vi "CCD spectrum processing_Shaowei-v4.vi"() -> ()   [LabVIEW 2012]
uses:
  <vilib>/Utility/file.llb/Read From Spreadsheet File (DBL).vi
panel:
  in  "save 2":bool
  in  "save 1":bool
  in  "select 2":bool
  in  "select":bool
  in  "next 2":bool
  in  "next":bool
  in  "previous 2":bool
  in  "previous":bool
  in  "Do it":bool
  out "?":path
  out "?":path
  out "Spec2 File name":string
  out "Spec1 File name":string
  in  "window switch":bool
  out "Spectrum 2":cluster{"Y":dbl[], "Y":dbl[]}[](graph)
  in  "?":bool=TRUE
  in  "?":bool
  out "Y":sgl
  out "X":sgl
  out "MIN":dbl
  out "MAX":dbl
  out "Spectrum 1":cluster{"Y":dbl[], "Y":dbl[]}[](graph)
  in  "file switch":bool
  out "?":ext=1340.0
  in  "cosmic ray removal":bool
  in  "?":i32(ring)=1 items=["nm"=1, "eV"=2, "cm-1"=3, "Pixel #"=4]
  # "Input File"
  # "1 File"
  # "2 Files"
  # "1st"
  # "2nd"
  # "Active Window"
  # "#1"
  # "#2"
  # "Save As"
  # "# of Pixel"
  # "X unit"
  # "Cosmic Ray Removal"
  # "NO"
  # "YES"
  # "Value"
  # "Position"
  # "Output Setting"
  # "Descending"
  # "Sort Data by X"
  # "Save As"
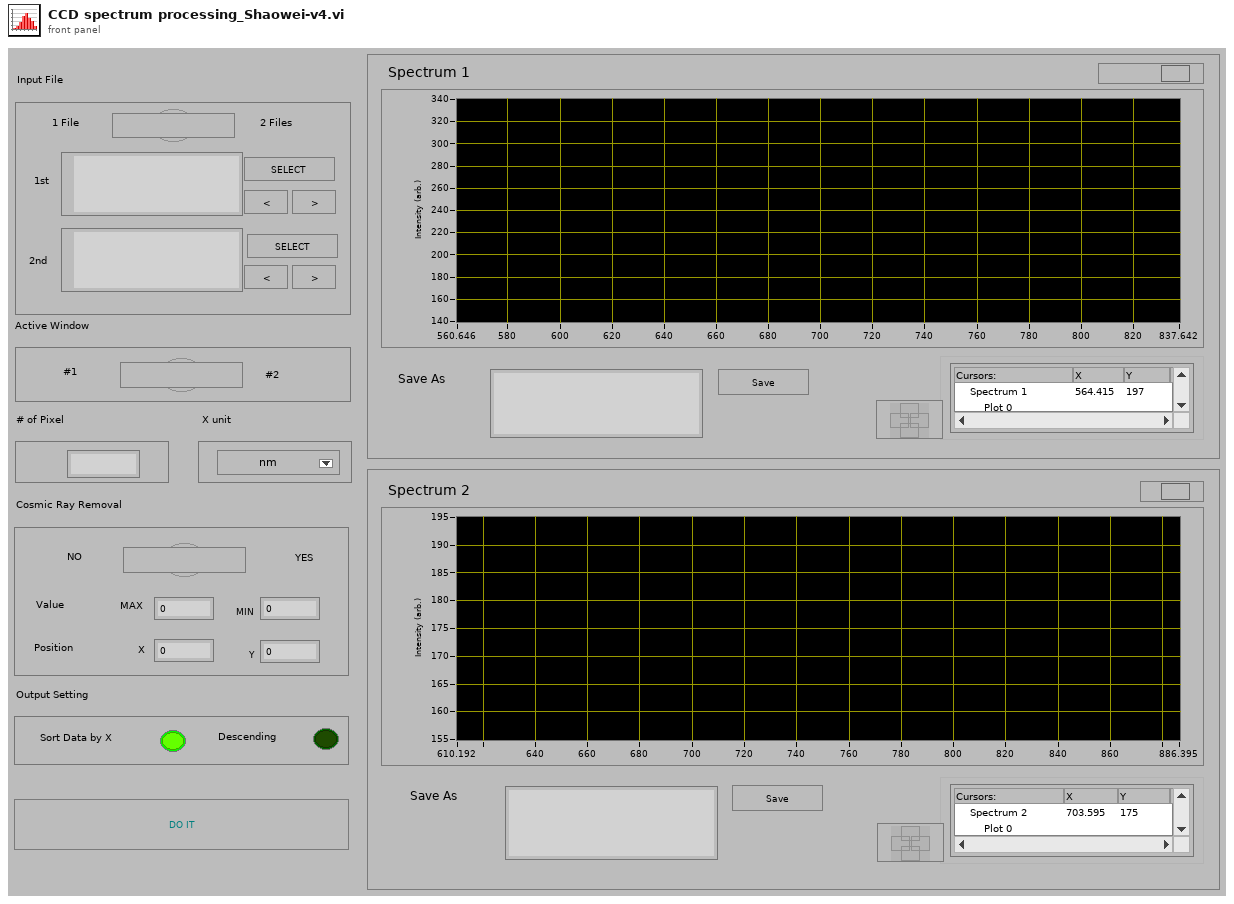
[diagram p1: front panel]
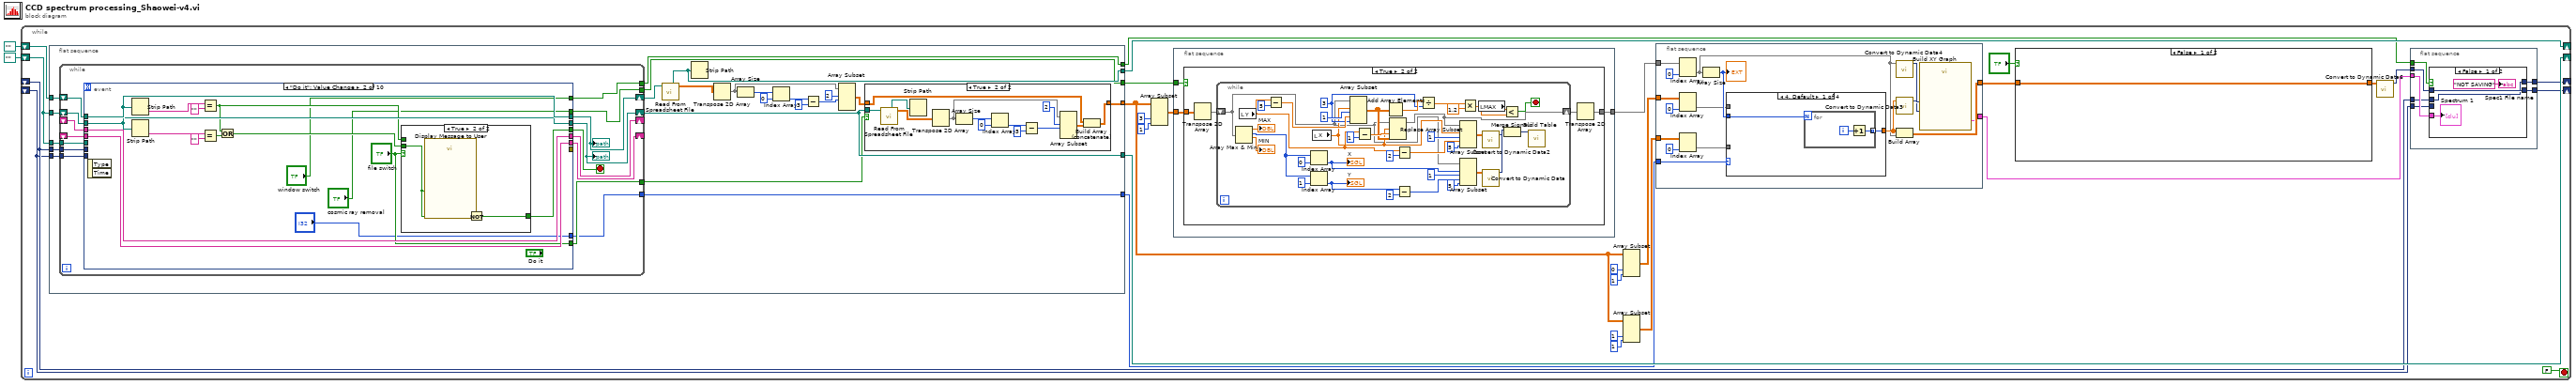
[diagram p0: block diagram]
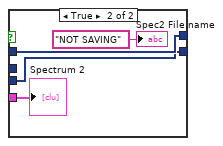
[diagram p2: hidden frame]
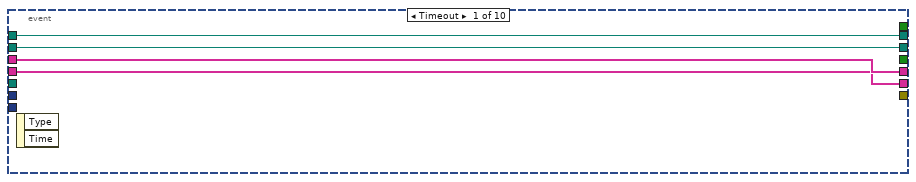
[diagram p3: hidden frame]
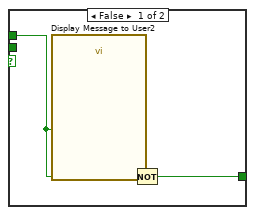
[diagram p4: hidden frame]
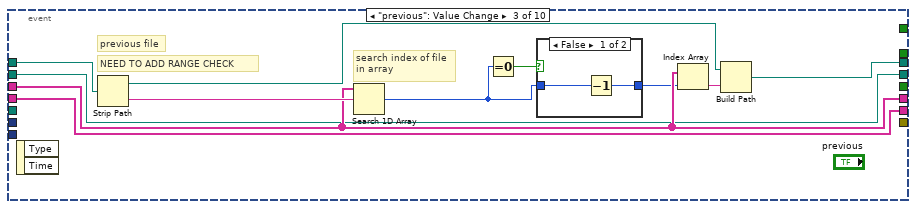
[diagram p5: hidden frame]
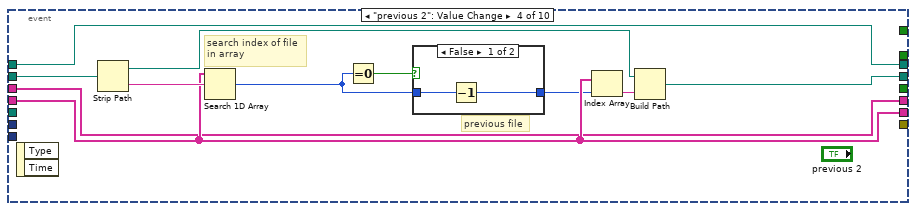
[diagram p7: hidden frame]
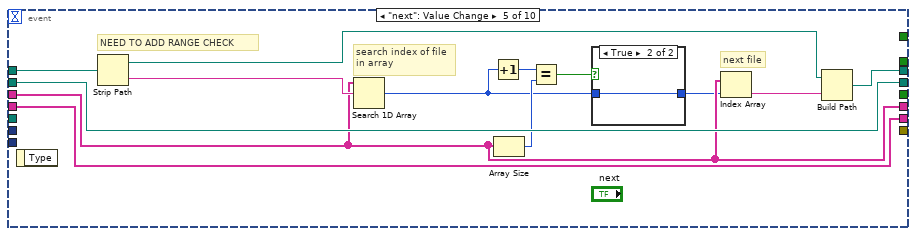
[diagram p9: hidden frame]
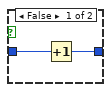
[diagram p10: hidden frame]
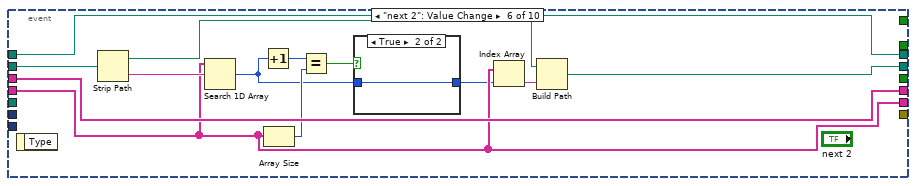
[diagram p11: hidden frame]
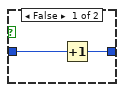
[diagram p12: hidden frame]
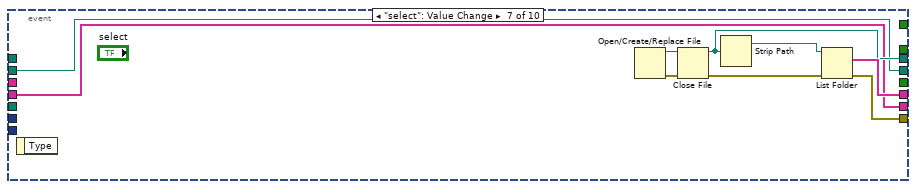
[diagram p13: hidden frame]
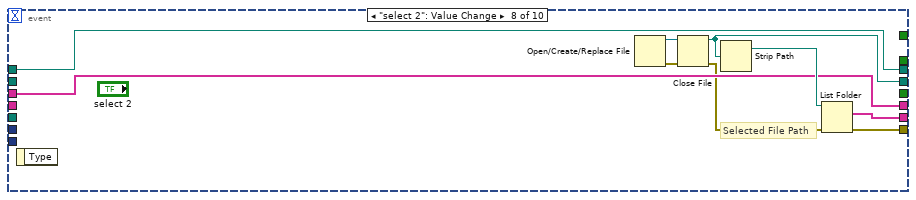
[diagram p14: hidden frame]
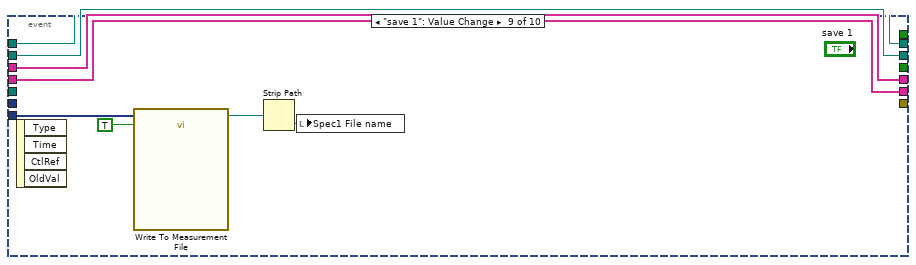
[diagram p15: hidden frame]
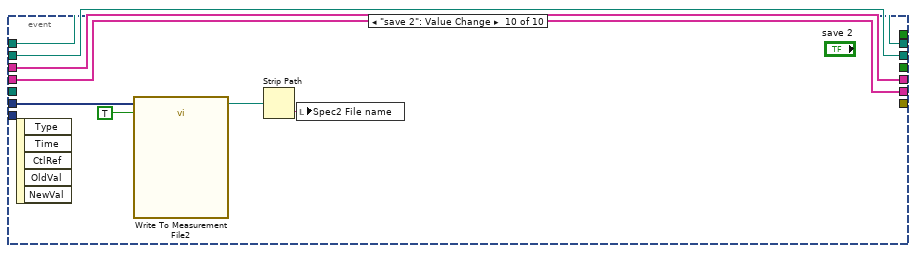
[diagram p16: hidden frame]
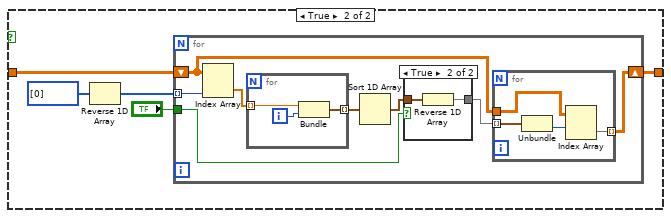
[diagram p18: hidden frame]
diagram:
  n1 = while {
    shift-right: [w22] -> _
    shift-left: path "" ("new file path (Not A Path if cancelled)") -> [w23]
    shift-right: [w21] -> _
    shift-left: path "" ("path") -> [w3]
    shift-right: [w7] -> _
    shift-left: _ -> [w4]
    shift-right: [w6] -> _
    shift-left: _ -> [w5]
    stop <- FALSE ("stop 2") stop-if-true
    n2 = flat-sequence {
      tunnel: [w66] -> w10
      tunnel: w23 -> [w64]
      tunnel: w3 -> [w63]
      tunnel: [w62] -> w22
      tunnel: [w61] -> w21
      tunnel: [w59] -> w20
      tunnel: [w58] -> w19
      tunnel: [w57] -> w18
      tunnel: w5 -> [w56]
      tunnel: w4 -> [w55]
      tunnel: w3 -> [w46]
      frame #0 {
        n3 = while {
          shift-right: [w82] -> _
          shift-left: _ -> [w81]
          shift-right: [w83] -> w65
          shift-left: w64 -> [w80]
          shift-right: [w79] -> w61
          shift-left: w63 -> [w78]
          shift-right: [w77] -> _
          shift-left: _ -> [w76]
          tunnel: [w71] -> w60
          tunnel: [w69] -> w59
          tunnel: [w68] -> w58
          tunnel: [w70] -> w57
          tunnel: w56 -> [w74]
          tunnel: w55 -> [w73]
          tunnel: w46 -> [w72]
          stop <- w75 stop-if-true
          n4 = event shown="[1] \"Do it\": Value Change" {
            selector: _ -> [_ _ _ _ _ _ _ _ _ _]
            dyn-events: _ -> [_ _ _ _ _ _ _ _ _ _]
            timeout: _ -> [_ _ _ _ _ _ _ _ _ _]
            tunnel: [_ w95 _ _ _ _ _ _ _ _] -> w75
            tunnel: [w86 w101 w113 w122 w145 w153 w173 w181 w193 w201] -> w83
            tunnel: [w87 w103 w115 w127 w138 w161 w174 w180 w192 w200] -> w82
            tunnel: w81 -> [w87 w103 w115 w127 w138 w161 _ w180 w192 w200]
            tunnel: w80 -> [w86 w101 w118 w122 w144 w153 _ w181 w193 w201]
            tunnel: [w84 w96 w111 w123 w142 w154 w171 w183 w187 w196] -> w79
            tunnel: w78 -> [w84 w96 w111 w129 w142 w152 w171 _ w187 w196]
            tunnel: [w85 w102 w112 w128 w143 w157 w172 w182 w188 w197] -> w77
            tunnel: w76 -> [w85 w102 w112 w128 w143 w157 w172 _ w188 w197]
            tunnel: [_ _ _ _ _ _ w168 w177 _ _] -> _
            tunnel: w74 -> [_ _ _ _ _ _ _ _ _ w194]
            tunnel: w73 -> [_ _ _ _ _ _ _ _ w186 _]
            tunnel: w72 -> [_ _ _ _ _ _ _ _ _ _]
            tunnel: [_ "file switch" _ _ _ _ _ _ _ _] -> w71
            tunnel: [_ "window switch" _ _ _ _ _ _ _ _] -> w70
            tunnel: [_ "cosmic ray removal" _ _ _ _ _ _ _ _] -> w69
            tunnel: [_ "?" _ _ _ _ _ _ _ _] -> w68
            event Timeout {
              n5 = event-data() -> ()  [unwired: 1 in, 2 out]
            }
            event "Do it": Value Change {
              n6 = event-data() -> ()  [unwired: 1 in, 2 out]
              n7 = Strip Path(path=w101) -> (name=w100:string)  [unwired: 1 out]
              n8 = Strip Path(path=w96) -> (name=w98:string)  [unwired: 1 out]
              n9 = Equal?(x=w100, y="") -> (x = y?=w94:bool)
              n10 = Equal?(x=w98, y="") -> (x = y?=w93:bool)
              n11 = Or(x=w94, y=w93) -> (x .or. y?=w92:bool)
              n12 = case shown="True" "file switch" {
                tunnel: w94 -> [w104 _]
                tunnel: [w105 w107] -> w95
                tunnel: w92 -> [_ w106]
                frame False {
                  n13 = call "Display Message to User2"("Enable"=w104) -> ()  [unwired: 9 in, 2 out]
                  n14 = Not(x=w104) -> (.not. x?=w105:bool)
                }
                frame True {
                  n15 = call "Display Message to User"("Enable"=w106) -> ()  [unwired: 9 in, 2 out]
                  n16 = Not(x=w106) -> (.not. x?=w107:bool)
                }
              }
            }
            event "previous": Value Change {
              # "NEED TO ADD RANGE CHECK"
              # "previous file"
              # "search index of file\nin array"
              n17 = event-data() -> ()  [unwired: 1 in, 2 out]
              n18 = Strip Path(path=w118) -> (stripped path=w116:path, name=w117:string)
              n19 = Search 1D Array(1D array=w115, element=w117) -> (index of element=w109:i32)  [unwired: 1 in]
              n20 = Equal To 0?(x=w109) -> (x = 0?=w110:bool)
              n21 = case shown="False" w110 {
                tunnel: w109 -> [w120 w121]
                tunnel: [w119 w121] -> w108
                frame False {
                  n22 = Decrement(x=w120) -> (x-1=w119:i32)
                }
                frame True {
                }
              }
              n23 = Index Array(array=w115, index=w108) -> (element=w114:string)
              n24 = Build Path(base path=w116, name or relative path=w114) -> (appended path=w113:path)
            }
            event "previous 2": Value Change {
              # "previous file"
              # "search index of file\nin array"
              n25 = event-data() -> ()  [unwired: 1 in, 2 out]
              n26 = Strip Path(path=w129) -> (stripped path=w131:path, name=w132:string)
              n27 = Search 1D Array(1D array=w128, element=w132) -> (index of element=w125:i32)  [unwired: 1 in]
              n28 = Equal To 0?(x=w125) -> (x = 0?=w126:bool)
              n29 = case shown="False" w126 {
                tunnel: w125 -> [w134 w135]
                tunnel: [w133 w135] -> w124
                frame False {
                  n30 = Decrement(x=w134) -> (x-1=w133:i32)
                }
                frame True {
                }
              }
              n31 = Index Array(array=w128, index=w124) -> (element=w130:string)
              n32 = Build Path(base path=w131, name or relative path=w130) -> (appended path=w123:path)
            }
            event "next": Value Change {
              # "NEED TO ADD RANGE CHECK"
              # "next file"
              # "search index of file\nin array"
              n33 = event-data() -> ()  [unwired: 1 in, 1 out]
              n34 = Strip Path(path=w144) -> (stripped path=w147:path, name=w148:string)
              n35 = Search 1D Array(1D array=w138, element=w148) -> (index of element=w137:i32)  [unwired: 1 in]
              n36 = Increment(x=w137) -> (x+1=w139:i32)
              n37 = Array Size(array=w138) -> (size(s)=w141:i32)
              n38 = Equal?(x=w139, y=w141) -> (x = y?=w140:bool)
              n39 = case shown="True" w140 {
                tunnel: w137 -> [w150 w151]
                tunnel: [w149 w151] -> w136
                frame False {
                  n40 = Increment(x=w150) -> (x+1=w149:i32)
                }
                frame True {
                }
              }
              n41 = Index Array(array=w138, index=w136) -> (element=w146:string)
              n42 = Build Path(base path=w147, name or relative path=w146) -> (appended path=w145:path)
            }
            event "next 2": Value Change {
              n43 = event-data() -> ()  [unwired: 1 in, 1 out]
              n44 = Strip Path(path=w152) -> (stripped path=w163:path, name=w164:string)
              n45 = Search 1D Array(1D array=w157, element=w164) -> (index of element=w156:i32)  [unwired: 1 in]
              n46 = Increment(x=w156) -> (x+1=w158:i32)
              n47 = Array Size(array=w157) -> (size(s)=w160:i32)
              n48 = Equal?(x=w158, y=w160) -> (x = y?=w159:bool)
              n49 = case shown="True" w159 {
                tunnel: w156 -> [w166 w167]
                tunnel: [w165 w167] -> w155
                frame False {
                  n50 = Increment(x=w166) -> (x+1=w165:i32)
                }
                frame True {
                }
              }
              n51 = Index Array(array=w157, index=w155) -> (element=w162:string)
              n52 = Build Path(base path=w163, name or relative path=w162) -> (appended path=w154:path)
            }
            event "select": Value Change {
              n53 = event-data() -> ()  [unwired: 1 in, 1 out]
              n54 = Open/Create/Replace File() -> (refnum out=w176:refnum<file>, error out=w170:errorcluster)  [unwired: 6 in, 1 out]
              n55 = Close File(refnum=w176, error in=w170) -> (path=w173:path, error out=w169:errorcluster)
              n56 = Strip Path(path=w173) -> (stripped path=w175:path)  [unwired: 1 out]
              n57 = List Folder(path=w175, error in=w169) -> (filenames=w174:string[], error out=w168:errorcluster)  [unwired: 2 in, 2 out]
            }
            event "select 2": Value Change {
              # "Selected File Path"
              n58 = event-data() -> ()  [unwired: 1 in, 1 out]
              n59 = Open/Create/Replace File() -> (refnum out=w185:refnum<file>, error out=w179:errorcluster)  [unwired: 6 in, 1 out]
              n60 = Close File(refnum=w185, error in=w179) -> (path=w183:path, error out=w178:errorcluster)
              n61 = Strip Path(path=w183) -> (stripped path=w184:path)  [unwired: 1 out]
              n62 = List Folder(path=w184, error in=w178) -> (filenames=w182:string[], error out=w177:errorcluster)  [unwired: 2 in, 2 out]
            }
            event "save 1": Value Change {
              n63 = event-data() -> ()  [unwired: 1 in, 4 out]
              n64 = call "Write To Measurement File"("Signals"=w186, "Reset"=TRUE) -> ("Filename Out"=w191:path)  [unwired: 15 in, 2 out]
              n65 = Strip Path(path=w191) -> (name=w189:string)  [unwired: 1 out]
              n66 = local write "Spec1 File name"(w189) -> ()
            }
            event "save 2": Value Change {
              n67 = event-data() -> ()  [unwired: 1 in, 5 out]
              n68 = call "Write To Measurement File2"("Signals"=w194, "Reset"=TRUE) -> ("Filename Out"=w199:path)  [unwired: 15 in, 2 out]
              n69 = Strip Path(path=w199) -> (name=w195:string)  [unwired: 1 out]
              n70 = local write "Spec2 File name"(w195) -> ()
            }
          }
          "?" <- w83
          "?" <- w79
        }
        n71 = call-poly <vilib>:"Read From Spreadsheet File.vi"("file path (dialog if empty)"=w65) -> ("all rows"=w67:dbl[][], "new file path (Not A Path if cancelled)"=w62:path)  [unwired: 6 in, 3 out]
        n72 = Strip Path(path=w62) -> ()  [unwired: 2 out]
        n73 = Transpose 2D Array(2D array=w67) -> (transposed array=w48:dbl[][])
        n74 = Array Size(array=w48) -> (size(s)=w54:i32[])
        n75 = Index Array(array=w54, index=0) -> (element=w52:i32)
        n76 = Subtract(x=w52, y=3) -> (x-y=w50:i32)
        n77 = Array Subset(array=w48, index (row)=2 ("index"), length (row)=w50) -> (w47:dbl[][])  [unwired: 2 in]
        n78 = case shown="True" w60 {
          tunnel: w47 -> [w202 w212]
          tunnel: [w202 w211] -> w66
          tunnel: w61 -> [_ w213]
          frame False {
          }
          frame True {
            n79 = call-poly <vilib>:"Read From Spreadsheet File.vi"("file path (dialog if empty)"=w213) -> ("all rows"=w214:dbl[][], "new file path (Not A Path if cancelled)"=w215:path)  [unwired: 6 in, 3 out]
            n80 = Strip Path(path=w215) -> ()  [unwired: 2 out]
            n81 = Transpose 2D Array(2D array=w214) -> (transposed array=w204:dbl[][])
            n82 = Array Size(array=w204) -> (size(s)=w210:i32[])
            n83 = Index Array(array=w210, index=0) -> (element=w208:i32)
            n84 = Subtract(x=w208, y=3) -> (x-y=w206:i32)
            n85 = Array Subset(array=w204, index (row)=2 ("index"), length (row)=w206) -> (w203:dbl[][])  [unwired: 2 in]
            n86 = Build Array (concatenate)(w212, w203) -> (w211:dbl[][])
          }
        }
      }
    }
    n87 = Array Subset(array=w10, index (col)=3 ("index"), length (col)=1 ("length")) -> (w30:dbl[][])  [unwired: 2 in]
    n88 = flat-sequence {
      tunnel: w30 -> [w279]
      tunnel: w20 -> [w278]
      tunnel: [w277] -> w28
      frame #0 {
        n89 = case shown="True" w278 {
          tunnel: w279 -> [w280 w284]
          tunnel: [w280 w282] -> w277
          frame False {
          }
          frame True {
            n90 = Transpose 2D Array(2D array=w284) -> (transposed array=w283:dbl[][])
            n91 = while {
              shift-right: [w321] -> w281
              shift-left: w283 -> [w285]
              stop <- w300 stop-if-true
              w298 = 3
              n92 = Array Max & Min(array=w285) -> (max value=→"MAX":dbl, max index (indices)=w319:i32[], min value=→"MIN":dbl)  [unwired: 1 out]
              n93 = local read "Y"() -> (w287:sgl)
              n94 = Subtract(x=w287, y=5) -> (x-y=w315:sgl)
              n95 = Index Array(array=w319, index=0) -> (element=w292:i32)
              "X" <- w292
              n96 = Index Array(array=w319, index=1) -> (element=w291:i32)
              "Y" <- w291
              n97 = local read "X"() -> (w288:sgl)
              n98 = Array Subset(array=w285, index (row)=w288, length (row)=1, index (col)=w315, length (col)=w298) -> (w297:dbl[][])
              n99 = Subtract(x=w287, y=1) -> (x-y=w314:sgl)
              n100 = Add Array Elements(numeric array=w297) -> (sum=w299:dbl)
              n101 = Replace Array Subset(array=w285, new element=w297, index (row)=w288, index (col)=w314) -> (w321:dbl[][])
              n102 = Subtract(x=w287, y=2) -> (x-y=w310:sgl)
              n103 = Subtract(x=w291, y=2) -> (x-y=w305:i32)
              n104 = Divide(x=w299, y=w298) -> (x/y=w296:dbl)
              n105 = Array Subset(array=w321, index (row)=w288, length (row)=1, index (col)=w310, length (col)=5) -> (w308:dbl[][])
              n106 = Array Subset(array=w285, index (row)=w292, length (row)=1, index (col)=w305, length (col)=5) -> (w303:dbl[][])
              n107 = Multiply(x=w296, y=1.2) -> (x*y=w301:dbl)
              n108 = local read "MAX"() -> (w286:dbl)
              n109 = call "Convert to Dynamic Data2"("2D Array"=w308) -> ("Dynamic Data Type"=w293:dynamicdata)  [unwired: 3 in]
              n110 = call "Convert to Dynamic Data"("2D Array"=w303) -> ("Dynamic Data Type"=w295:dynamicdata)  [unwired: 3 in]
              n111 = Less?(x=w286, y=w301) -> (x < y?=w300:bool)
              n112 = Merge Signals(w295, w293) -> (w294:dynamicdata)
              n113 = call "Build Table"("Signals"=w294) -> ()  [unwired: 9 in, 2 out]
            }
            n114 = Transpose 2D Array(2D array=w281) -> (transposed array=w282:dbl[][])
          }
        }
      }
    }
    n115 = Array Subset(array=w10, index (col)=0 ("index"), length (col)=1 ("length")) -> (w9:dbl[][])  [unwired: 2 in]
    n116 = Array Subset(array=w10, index (col)=1 ("index"), length (col)=1 ("length")) -> (w13:dbl[][])  [unwired: 2 in]
    n117 = flat-sequence {
      tunnel: w28 -> [w255]
      tunnel: [w251] -> w27
      tunnel: w19 -> [w249]
      tunnel: [w247] -> w24
      tunnel: w13 -> [w245]
      tunnel: w9 -> [w241]
      frame #0 {
        n118 = Index Array(array=w255, index (col)=0) -> (element=w243:dbl[])  [unwired: 1 in]
        n119 = Index Array(array=w241, index (col)=0) -> (element=w240:dbl[])  [unwired: 1 in]
        n120 = Index Array(array=w245, index (col)=0) -> (element=w244:dbl[])  [unwired: 1 in]
        n121 = Array Size(array=w243) -> (size(s)=w248:i32)
        "?" <- w248
        n122 = case shown="4, Default" w249 {
          tunnel: w248 -> [w256 _ w263 w269]
          tunnel: [w257 w260 w262 w270] -> w252
          tunnel: w244 -> [_ w260 w261 w271]
          tunnel: w240 -> [_ _ _ _]
          frame 4, Default {
            n123 = for {
              N: w256 -> [_]
              tunnel: [w258] -> w257 mode=indexing
              i -> [w259]
              n124 = Increment(x=w259) -> (x+1=w258:i32)
            }
          }
          frame 1 {
          }
          frame 2 {
            n125 = for {
              N: w263 -> [_]
              tunnel: [w264] -> w262 mode=indexing
              tunnel: w261 -> [w268]
              i -> [w267]
              n126 = Index Array(array=w268, index=w267) -> (element=w266:dbl)
              n127 = Divide(x=1240.0, y=w266) -> (x/y=w264:dbl)
            }
          }
          frame 3 {
            n128 = for {
              N: w269 -> [_]
              tunnel: [w272] -> w270 mode=indexing
              tunnel: w271 -> [w276]
              i -> [w275]
              n129 = Index Array(array=w276, index=w275) -> (element=w274:dbl)
              n130 = Divide(x=10000000.0, y=w274) -> (x/y=w272:dbl)
            }
          }
        }
        n131 = call "Convert to Dynamic Data4"("Array"=w243) -> ("Dynamic Data Type"=w253:dynamicdata)  [unwired: 3 in]
        n132 = call "Convert to Dynamic Data3"("Array"=w252) -> ("Dynamic Data Type"=w254:dynamicdata)  [unwired: 3 in]
        n133 = Build Array(w252, w243) -> (w251:dbl[][])
        n134 = call "Build XY Graph"("Y Input"=w253, "X Input"=w254) -> ("XY Graph"=w247:cluster{"Y":dbl[], "Y":dbl[]}[])  [unwired: 8 in, 1 out]
      }
    }
    n135 = case shown="False" "?" {
      tunnel: w27 -> [w216 w218]
      tunnel: [w216 w217] -> w25
      frame False {
      }
      frame True {
        n136 = Reverse 1D Array(array=i32[] [0] ("Priority Columns (0)")) -> (reversed array=w220:i32[])
        n137 = for {
          shift-right: [w223] -> w217
          shift-left: w218 -> [w225]
          tunnel: w220 -> [w222] mode=indexing
          tunnel: "?" -> [w224]
          n138 = Index Array(array=w225, index (col)=w222) -> (element=w227:dbl[])  [unwired: 1 in]
          n139 = for {
            tunnel: w227 -> [w237] mode=indexing
            tunnel: [w239] -> w226 mode=indexing
            i -> [w238]
            n140 = Bundle(w237, w238) -> (w239:cluster{dbl, i32})  [unwired: 1 out]
          }
          n141 = Sort 1D Array(array=w226) -> (sorted array=w229:cluster{dbl, i32}[])
          n142 = case shown="True" w224 {
            tunnel: [w230 w231] -> w228
            tunnel: w229 -> [w230 w232]
            frame False {
            }
            frame True {
              n143 = Reverse 1D Array(array=w232) -> (reversed array=w231:cluster{dbl, i32}[])
            }
          }
          n144 = for {
            tunnel: w228 -> [w236] mode=indexing
            tunnel: w225 -> [w235]
            tunnel: [w233] -> w223 mode=indexing
            n145 = Unbundle(w236) -> (w234:i32)  [unwired: 1 out]
            n146 = Index Array(array=w235, index (row)=w234) -> (element=w233:dbl[])  [unwired: 1 in]
          }
        }
      }
    }
    n147 = call "Convert to Dynamic Data6"("2D Array"=w25) -> ("Dynamic Data Type"=w8:dynamicdata)  [unwired: 3 in]
    n148 = flat-sequence {
      tunnel: w24 -> [w37]
      tunnel: w18 -> [w36]
      tunnel: w8 -> [w35]
      tunnel: [w34] -> w7
      tunnel: [w33] -> w6
      tunnel: w5 -> [w32]
      tunnel: w4 -> [w31]
      frame #0 {
        n149 = case shown="False" w36 {
          tunnel: w37 -> [w41 w45]
          tunnel: w35 -> [w40 w44]
          tunnel: [w40 w43] -> w34
          tunnel: [w39 w44] -> w33
          tunnel: w32 -> [w39 _]
          tunnel: w31 -> [_ w43]
          frame False {
            "Spectrum 1" <- w41
            "Spec1 File name" <- "NOT SAVING"
          }
          frame True {
            "Spectrum 2" <- w45
            "Spec2 File name" <- "NOT SAVING" ("Spec1 File name")
          }
        }
      }
    }
  }
